vi "MSWord-UpdateBookmarks.vi"(8 "error in":errorcluster, 9 "Text Data":string[](array[string]), 11 "Bookmarks":string[](array[string])) -> (0 "error out":errorcluster)   [LabVIEW 2013]
panel:
  in  "Path":path=path "C:/Work Order Template/testing.docx"
  in  "Word._Application":refnum<k7>
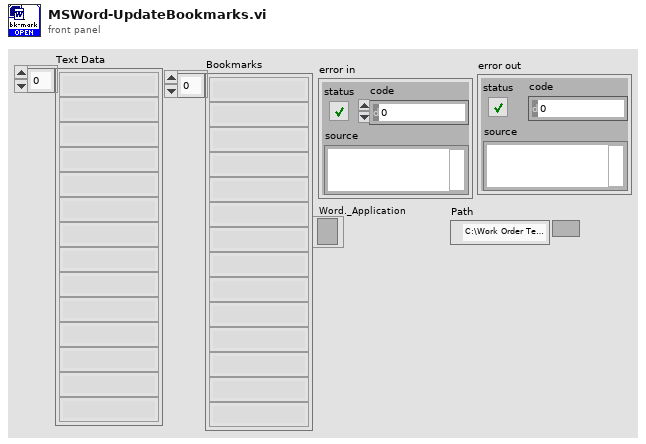
[diagram p1: front panel]
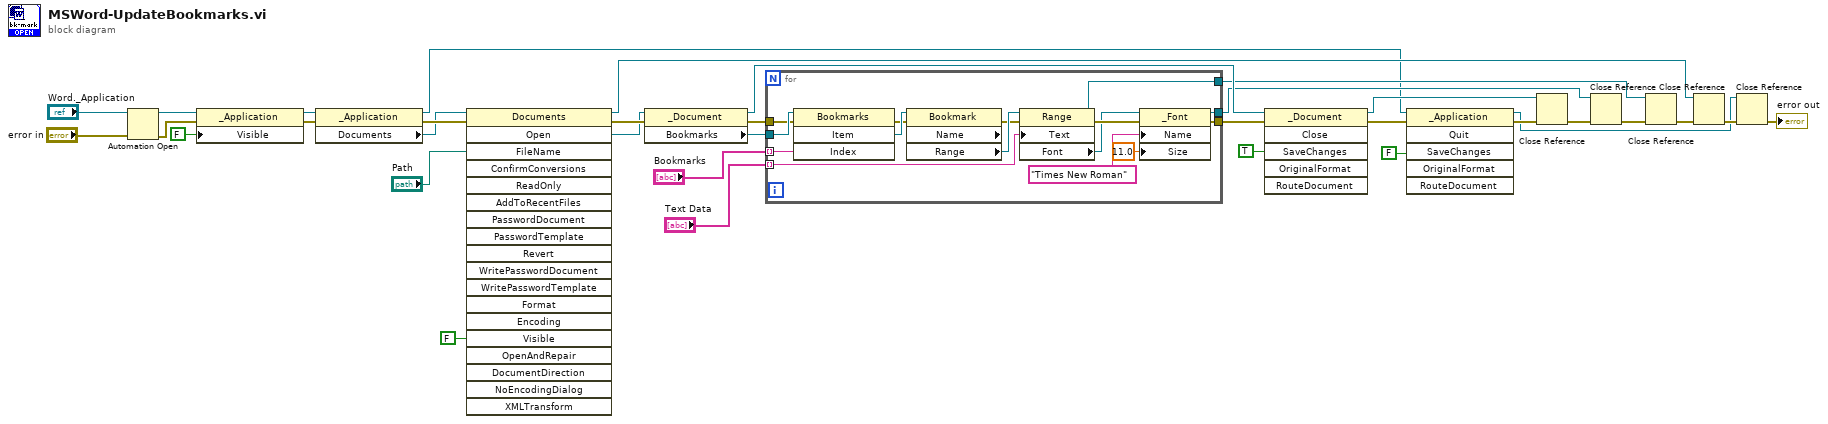
[diagram p0: block diagram]
diagram:
  n1 = Automation Open(error in (no error)="error in", Automation Refnum="Word._Application") -> (Automation Refnum=w29:refnum<k7>, error out=w7:errorcluster)  [unwired: 2 in]
  n2 = property class="_Application"(reference=w29, error in=w7, "Visible"=FALSE) -> (reference out=w30:refnum<k7>, error out=w31:errorcluster)
  n3 = property class="_Application"(reference=w30, error in=w31) -> (reference out=w3:refnum<k7>, error out=w21:errorcluster, "Documents"=w20:refnum<k7>)
  n4 = invoke class="Documents" method="Open"(reference=w20, error in=w21, "FileName"="Path", "Visible"=FALSE) -> (reference out=w12:refnum<k7>, error out=w24:errorcluster, "Open"=w23:refnum<k7>)  [unwired: 15 in, 16 out]
  n5 = property class="_Document"(reference=w23, error in=w24) -> (reference out=w33:refnum<k7>, error out=w18:errorcluster, "Bookmarks"=w25:refnum<k7>)
  n6 = for {
    tunnel: w25 -> [w49]
    tunnel: "Bookmarks" -> [w46] mode=indexing
    tunnel: w18 -> [w45]
    tunnel: "Text Data" -> [w42] mode=indexing
    tunnel: [w39] -> w16
    tunnel: [w38] -> w13
    tunnel: [w35] -> w8
    n7 = invoke class="Bookmarks" method="Item"(reference=w49, error in=w45, "Index"=w46) -> (error out=w47:errorcluster, "Item"=w48:refnum<k7>)  [unwired: 1 in, 2 out]
    n8 = property class="Bookmark" props=["Name", "Range"](reference=w48, error in=w47) -> (error out=w43:errorcluster, "Range"=w44:refnum<k7>)  [unwired: 2 out]
    n9 = property class="Range"(reference=w44, error in=w43, "Text"=w42) -> (reference out=w38:refnum<k7>, error out=w41:errorcluster, "Font"=w40:refnum<k7>)
    n10 = property class="_Font"(reference=w40, error in=w41, "Name"="Times New Roman", "Size"=sgl 11.0) -> (reference out=w35:refnum<k7>, error out=w39:errorcluster)
  }
  n11 = invoke class="_Document" method="Close"(reference=w33, error in=w16, "SaveChanges"=TRUE) -> (reference out=w14:refnum<k7>, error out=w5:errorcluster)  [unwired: 3 in, 4 out]
  n12 = invoke class="_Application" method="Quit"(reference=w3, error in=w5, "SaveChanges"=FALSE) -> (reference out=w2:refnum<k7>, error out=w4:errorcluster)  [unwired: 3 in, 4 out]
  n13 = Close Reference(reference=w14, error in (no error)=w4) -> (error out=w9:errorcluster)
  n14 = Close Reference(reference=w8, error in (no error)=w9) -> (error out=w6:errorcluster)
  n15 = Close Reference(reference=w13, error in (no error)=w6) -> (error out=w15:errorcluster)
  n16 = Close Reference(reference=w12, error in (no error)=w15) -> (error out=w26:errorcluster)
  n17 = Close Reference(reference=w2, error in (no error)=w26) -> (error out=→"error out":errorcluster)
